vi "OCR Control.vi"() -> ()   [LabVIEW 2014]
uses:
  Resources/Global.vi
  <vilib>/vision/NI_Vision_Development_Module.lvlib
panel:
  in  "Range":cluster{"Lower value":sgl, "Upper value":sgl}={"Lower value"=180.0, "Upper value"=255.0}
  in  "Number of Erosion":i32=2
  out "Command string":string
  out "State":string
  out "Land/TakeOff":bool
  out "Get Video Stream Error":errorcluster
  out "OCR":T1(plugin-control)
  out "Number of Lines":i32
  out "Read String":string
  in  "error in (no error)":errorcluster
  # "Do NOT run this VI. Instead run \"AR.Drone MAIN.vi\" and select the name of this VI in the dop-down menu at the Steup tab"
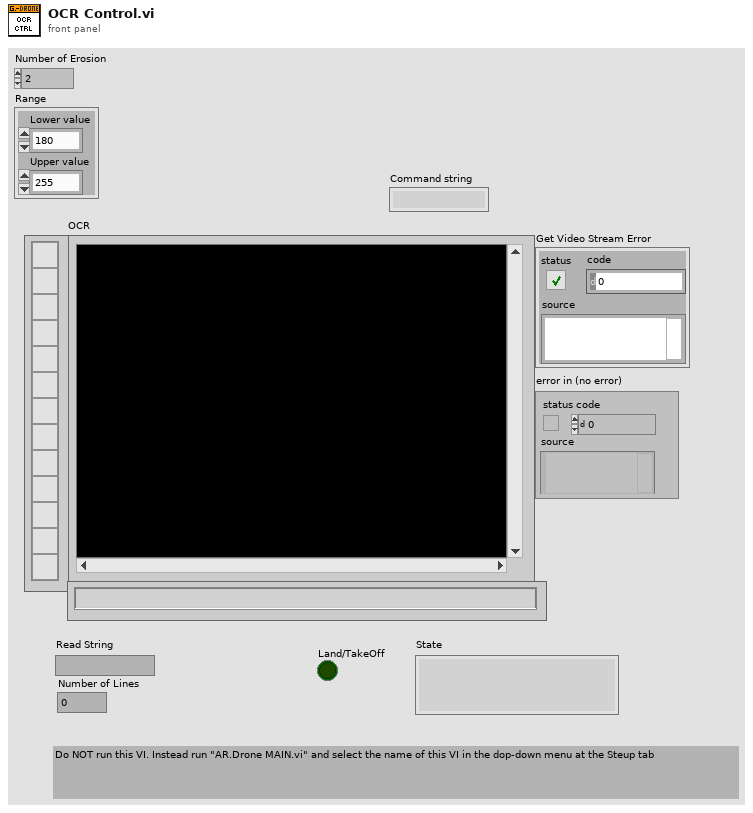
[diagram p1: front panel]
types:
  T1 = typedef "IMAQ Image.ctl" = refnum<image>
  T2 = typedef "Image Type" = u32
  T3 = typedef "IMAQ OCR Session.ctl" = refnum<k1>
  T4 = cluster{"Desired Font (Application)":enum16{"User-specified Font", "Application Font", "System Font", "Dialog Font"}, "[User-specified Font]":cluster{"Font Name":string, "Size":i16, "Strikeout?":bool, "Italic?":bool, "Underline?":bool, "Outline?":bool, "Shadow?":bool, "Bold?":bool, "Rotation Angle":dbl}, "Horizontal Alignment":i16, "Vertical Alignment":i16}
  T5 = cluster{"Left":dbl, "Top":dbl, "Right":dbl, "Bottom":dbl}
  T6 = cluster{"Left":dbl, "Top":dbl, "Right":dbl, "Bottom":dbl, dbl}
  T7 = typedef "ROI Descriptor" = cluster{"Global Rectangle":i32[], "Contours":cluster{"ID":enum32{"External", "Internal"}, "Type":u32, "Coordinates":i32[]}[]}
  T8 = cluster{"Global Rectangle":i32[], "Contours":cluster{"ID":enum32{"External", "Internal"}, "Type":u32, "Coordinates":i32[]}[]}
  T9 = typedef "Control cluster.ctl" = cluster{"Roll":sgl, "Pitch":sgl, "Vertical Speed":sgl, "Yaw Speed":sgl}
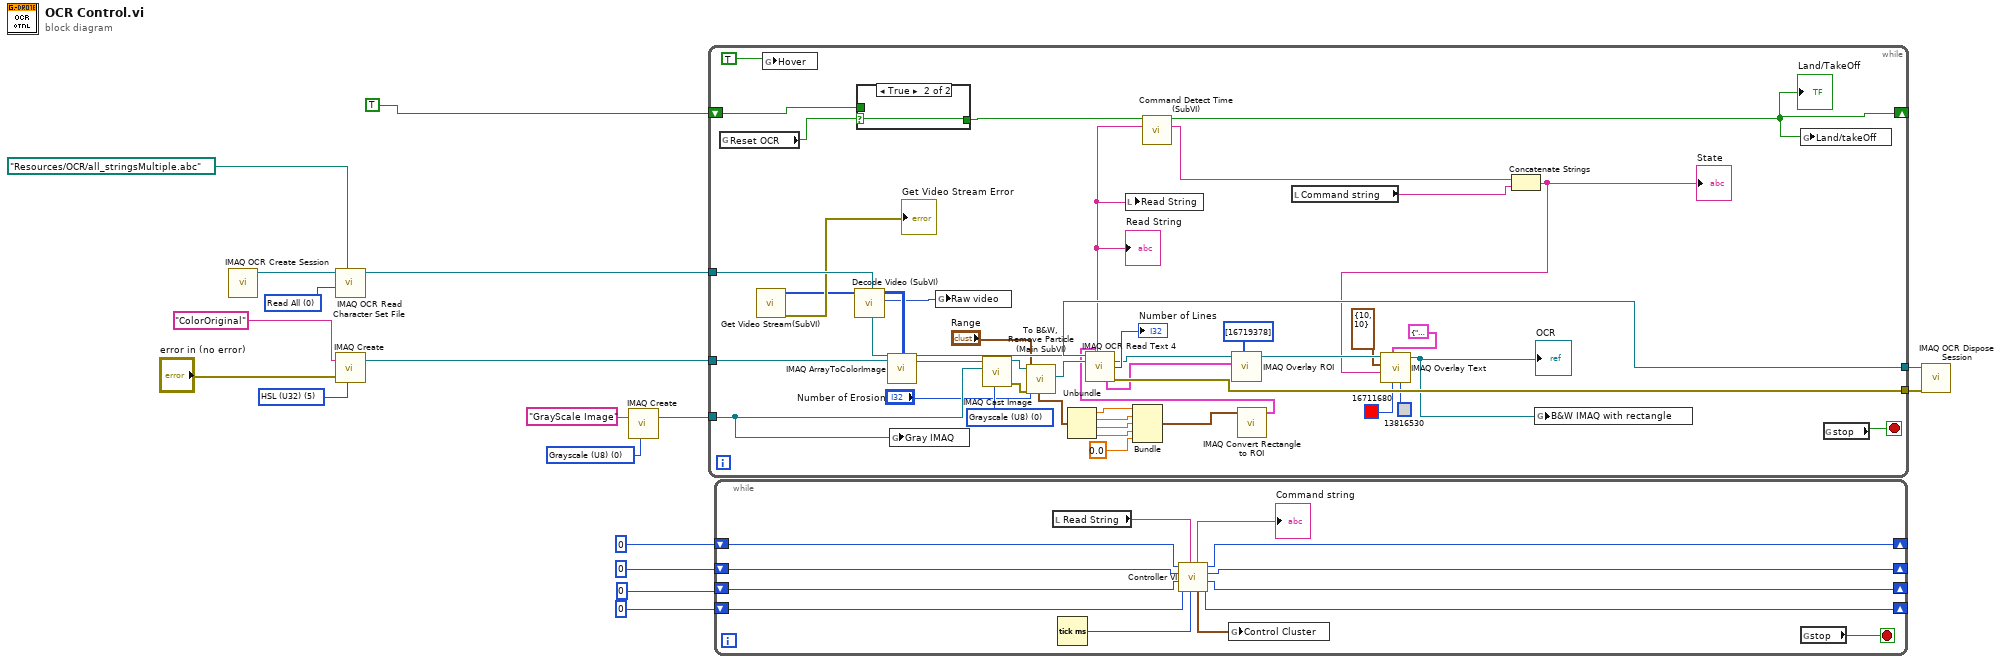
[diagram p0: block diagram]
diagram:
  w1 = 0 items=["Read All", "Read Character Set Only", "Read Properties Only"] ("Read Options")
  w4 = T2 0 items=["Grayscale (U8)", "Grayscale (I16)", "Grayscale (SGL)", "Complex (CSG)", "RGB (U32)", "HSL (U32)", "RGB (U64)", "Grayscale (U16)"] ("Image Type")
  w18 = T2 5 items=["Grayscale (U8)", "Grayscale (I16)", "Grayscale (SGL)", "Complex (CSG)", "RGB (U32)", "HSL (U32)", "RGB (U64)", "Grayscale (U16)"] ("Image Type")
  n1 = call "IMAQ OCR Create Session"() -> ("IMAQ OCR Session"=w13:T3)  [unwired: 10 in, 1 out]
  n2 = call "IMAQ OCR Read Character Set File"("File Path"=path "Resources/OCR/all_stringsMultiple.abc", "Read Options"=w1, "IMAQ OCR Session"=w13) -> ("IMAQ OCR Session (dup)"=w12:T3)  [unwired: 6 in, 2 out]
  n3 = call "IMAQ Create"("Image Name"="ColorOriginal", "Image Type"=w18, "error in (no error)"="error in (no error)") -> ("New Image"=w17:T1)  [unwired: 2 in, 1 out]
  n4 = call "IMAQ Create"("Image Name"="GrayScale Image", "Image Type"=w4) -> ("New Image"=w2:T1)  [unwired: 3 in, 1 out]
  n5 = while {
    tunnel: w17 -> [w53]
    tunnel: [w61] -> w15
    tunnel: [w60] -> w14
    tunnel: w12 -> [w59]
    shift-right: [w49] -> _
    shift-left: TRUE -> [w51]
    tunnel: w2 -> [w33]
    stop <- w47 stop-if-true
    w62 = T2 0 items=["Grayscale (U8)", "Grayscale (I16)", "Grayscale (SGL)", "Complex (CSG)", "RGB (U32)", "HSL (U32)", "RGB (U64)", "Grayscale (U16)"] ("Image Type")
    n6 = global read "Global.vi" "Reset OCR"() -> (w32:bool)
    n7 = call "Get Video Stream(SubVI).vi"() -> ("error out"=→"Get Video Stream Error":errorcluster, "ImgData"=w44:u8[])  [unwired: 10 in]
    n8 = global write "Global.vi" "Hover"(TRUE ("Hover")) -> ()
    n9 = call "Decode Video (SubVI).vi"("ImgData"=w44) -> ("new picture"=w42:picture, "Array"=w43:u32[][])  [unwired: 9 in]
    n10 = case shown="True" w32 {
      selector: w32 -> [_ w64]
      tunnel: w51 -> [w63 _]
      tunnel: [w63 w64] -> w50
      frame False {
      }
      frame True {
      }
    }
    n11 = call "IMAQ ArrayToColorImage"("Image Pixels (U32)"=w43, "Image"=w53) -> ("Image Out"=w54:T1)  [unwired: 3 in, 1 out]
    n12 = global write "Global.vi" "Gray IMAQ"(w33) -> ()
    n13 = global write "Global.vi" "Raw video"(w42) -> ()
    n14 = call "IMAQ Cast Image"("Image Type"=w62, "Image Dst"=w33, "Image Src"=w54) -> ("error out"=w31:errorcluster, "Image Dst Out"=w30:T1)  [unwired: 7 in]
    n15 = call "To B&W, Remove Particle (Main SubVI).vi"("error in (no error)"=w31, "Range"="Range", "Number of Erosion"="Number of Erosion", "Refnum in"=w30) -> ("Image Out"=w29:T1, "Cluster"=w25:T5)  [unwired: 1 in, 5 out]
    n16 = Unbundle(w25) -> ("Left"=w24:dbl, "Top"=w23:dbl, "Right"=w22:dbl, "Bottom"=w21:dbl)
    n17 = Bundle("Left"=w24, "Top"=w23, "Right"=w22, "Bottom"=w21, 0.0) -> (w26:T6)  [unwired: 1 in]
    n18 = call "IMAQ Convert Rectangle to ROI"("Rectangle"=w26) -> ("ROI Descriptor"=w19:T7)  [unwired: 8 in, 1 out]
    n19 = call "IMAQ OCR Read Text 4"("IMAQ OCR Session"=w59, "ROI Descriptor"=w19, "Image"=w29) -> ("IMAQ OCR Session (dup)"=w60:T3, "Image (dup)"=w55:T1, "Number of Lines"=→"Number of Lines":i32, "Read String"=w46:string, "ROI Bounding Characters"=w57:T8, "error out"=w61:errorcluster)  [unwired: 6 in, 1 out]
    "Read String" <- w46
    n20 = local write "Read String"(w46) -> ()
    n21 = call "Command Detect Time (SubVI).vi"("Read String"=w46, "Boolean in"=w50) -> ("String"=w45:string, "Boolean out"=w49:bool)  [unwired: 8 in]
    "Land/TakeOff" <- w49
    n22 = call "IMAQ Overlay ROI"("Colors (Green)"=u32[] [16719378], "ROI Descriptor"=w57, "Image"=w55) -> ("Image Out"=w41:T1)  [unwired: 7 in, 1 out]
    n23 = local read "Command string"() -> (w34:string)
    n24 = Concatenate Strings(w45, w34) -> (w39:string)
    "State" <- w39
    n25 = call "IMAQ Overlay Text"("BG Color (Transparent)"=u32 13816530, "Text Color (black)"=u32 16711680, "Font, Size & Style"=T4 {"Desired Font (Application)"=enum."User-specified Font", "[User-specified Font]"={"Font Name"="Calibri", "Size"=30, "Strikeout?"=FALSE, "Italic?"=FALSE, "Underline?"=FALSE, "Outline?"=TRUE, "Shadow?"=TRUE, "Bold?"=TRUE, "Rotation Angle"=0.0}, "Horizontal Alignment"=0, "Vertical Alignment"=1}, "String"=w39, "Origin"=cluster{"X":i32, "Y":i32} {"X"=10, "Y"=10}, "Image"=w41) -> ("Image Out"=w40:T1)  [unwired: 4 in, 1 out]
    "OCR" <- w40
    n26 = global write "Global.vi" "B&W IMAQ with rectangle"(w40) -> ()
    n27 = global write "Global.vi" "Land/takeOff"(w49) -> ()
    n28 = global read "Global.vi" "stop"() -> (w47:bool)
  }
  n29 = while {
    shift-right: [w69] -> _
    shift-left: u32 0 ("millisecond timer value") -> [w65]
    shift-right: [w71] -> _
    shift-left: u32 0 ("millisecond timer value") -> [w67]
    shift-right: [w70] -> _
    shift-left: u32 0 ("millisecond timer value") -> [w66]
    shift-right: [w72] -> _
    shift-left: u32 0 ("millisecond timer value") -> [w68]
    stop <- w77 stop-if-true
    n30 = local read "Read String"() -> (w74:string)
    n31 = Tick Count (ms)() -> (millisecond timer value=w75:u32)
    n32 = call "Controller VI.vi"("Current Time In"=w75, "Read String"=w74, "Down Detect Time In"=w65, "Up Detect Time In"=w66, "Left Detect Time In"=w67, "Right Detect Time In"=w68) -> ("Down Detect Time Out"=w69:u32, "Up Detect Time Out"=w70:u32, "Left Detect Time Out"=w71:u32, "Right detect Time Out"=w72:u32, "Control Cluster"=w76:T9, "Command string"=→"Command string":string)
    n33 = global write "Global.vi" "Control Cluster"(w76) -> ()
    n34 = global read "Global.vi" "stop"() -> (w77:bool)
  }
  n35 = call "IMAQ OCR Dispose Session"("error in (no error)"=w15, "IMAQ OCR Session"=w14) -> ()  [unwired: 9 in, 1 out]
